vi "285A_Update.vi"(8 "错误输入（无错误）":errorcluster, 11 "VISA资源名称":refnum<visa-resource-name>) -> (0 "error out":errorcluster, 3 "VISA资源名称 2":refnum<visa-resource-name>)   [LabVIEW 2016]
panel:
  out "Z":dbl
  out "Y":dbl
  out "X":dbl
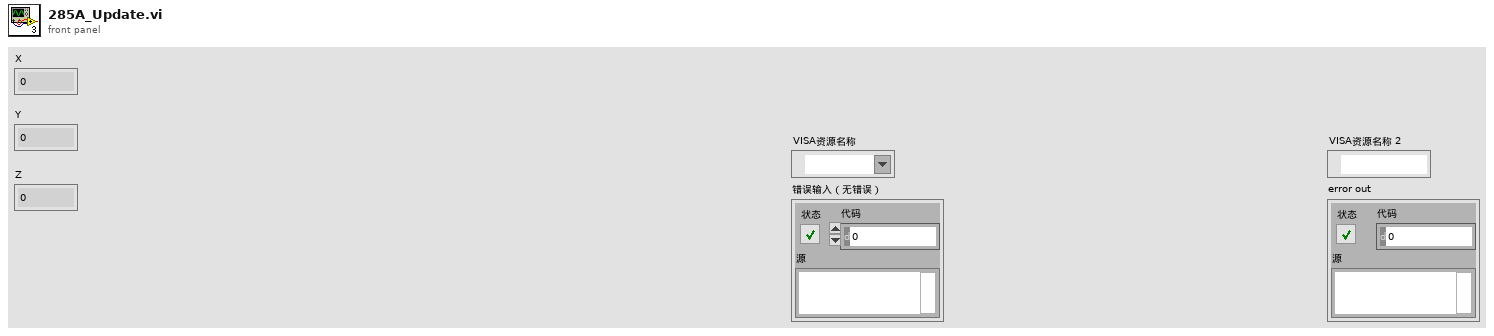
[diagram p1: front panel]
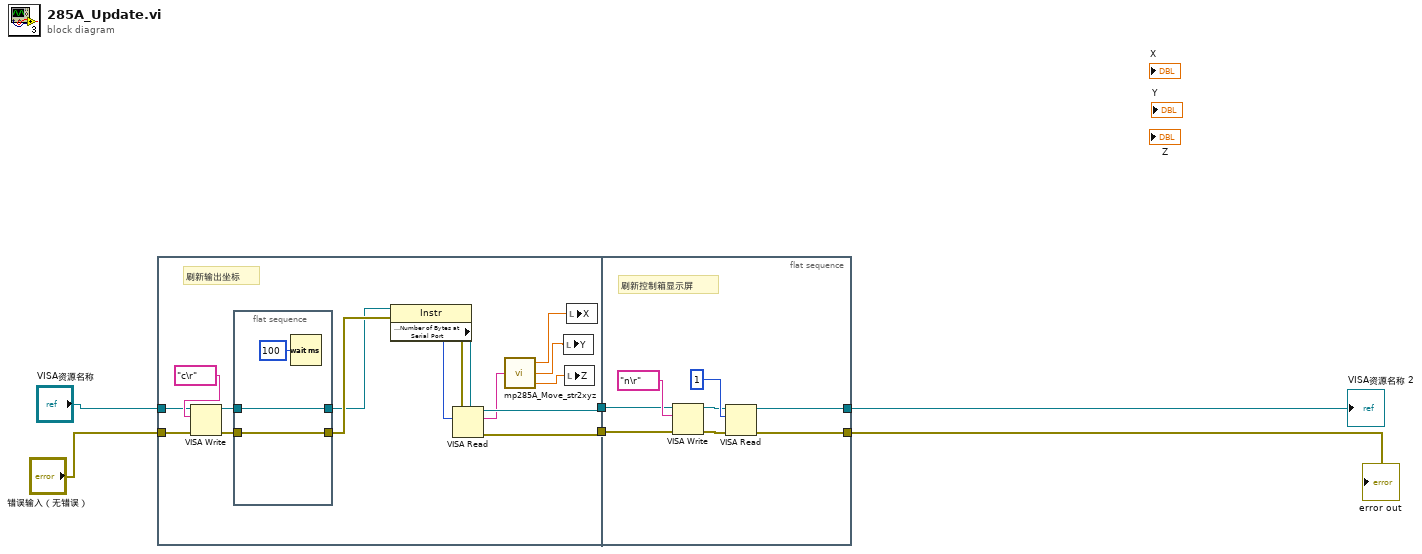
[diagram p0: block diagram]
diagram:
  n1 = flat-sequence {
    tunnel: [w11] -> w6
    tunnel: [w10] -> w5
    tunnel: "VISA资源名称" -> [w8]
    tunnel: "错误输入（无错误）" -> [w7]
    tunnel: [w30] -> w4
    tunnel: [w29] -> w3
    tunnel: w6 -> [w27]
    tunnel: w5 -> [w26]
    frame #0 {
      # "刷新输出坐标"
      n2 = VISA Write ("VISA写入")(VISA resource name=w8, write buffer="c\r" ("写入缓冲区"), error in (no error)=w7) -> (VISA resource name out=w19:refnum<visa-resource-name>, error out=w20:errorcluster)  [unwired: 1 out]
      n3 = flat-sequence {
        tunnel: w19 -> [w24]
        tunnel: w20 -> [w23]
        tunnel: [w24] -> w21
        tunnel: [w23] -> w22
        frame #0 {
          n4 = Wait (ms)(milliseconds to wait=u32 100 ("等待时间（毫秒）")) -> ()  [unwired: 1 out]
        }
      }
      n5 = property class="Instr"(reference=w21, error in=w22) -> (reference out=w14:refnum<visa-resource-name>, error out=w13:errorcluster, "Serial Settings:Number of Bytes at Serial Port"=w15:u32)
      n6 = VISA Read(VISA resource name=w14, byte count=w15, error in (no error)=w13) -> (VISA resource name out=w11:refnum<visa-resource-name>, read buffer=w9:string, error out=w10:errorcluster)  [unwired: 1 out]
      n7 = call "mp285A_Move_str2xyz.vi"("字符串"=w9) -> ("X轴"=w16:dbl, "Y轴"=w17:dbl, "Z轴"=w18:dbl)
      n8 = local write "Y"(w17) -> ()
      n9 = local write "Z"(w18) -> ()
      n10 = local write "X"(w16) -> ()
    }
    frame #1 {
      # "刷新控制箱显示屏"
      n11 = VISA Write ("VISA写入")(VISA resource name=w27, write buffer="n\r" ("写入缓冲区"), error in (no error)=w26) -> (VISA resource name out=w32:refnum<visa-resource-name>, error out=w31:errorcluster)  [unwired: 1 out]
      n12 = VISA Read(VISA resource name=w32, byte count=u32 1 ("字节总数"), error in (no error)=w31) -> (VISA resource name out=w30:refnum<visa-resource-name>, error out=w29:errorcluster)  [unwired: 2 out]
    }
  }
  "VISA资源名称 2" <- w4
  "error out" <- w3
